vi "Configure Warm Up Supply.vi"(0 "VISA resource name":refnum<visa-resource-name>, 5 "Unpowered Analog Output (3:3)":u16(ring)=3 items=["3"=3, "4"=4], 7 "Warm Up Control  (0:Auto Off)":u16(ring) items=["Auto Off", "Continuous"], 9 "Warm Up Percentage (0.00)":dbl format="%.2f", 11 "error in (no error)":errorcluster) -> (4 "VISA resource name out":refnum<visa-resource-name>, 15 "error out":errorcluster)   [LabVIEW 2019, in "Lake Shore 336.lvlib"]
doc: "This VI configures the Unpowered Analog Output when the mode is set to warm up supply. Warm up supply mode is designed for controlling an external power supply used for rapidly increasing the temperature in order to change samples."
uses:
  Lake Shore 336.lvlib
  Instance           1 32Saved   Configure Warm Up Supply .vi
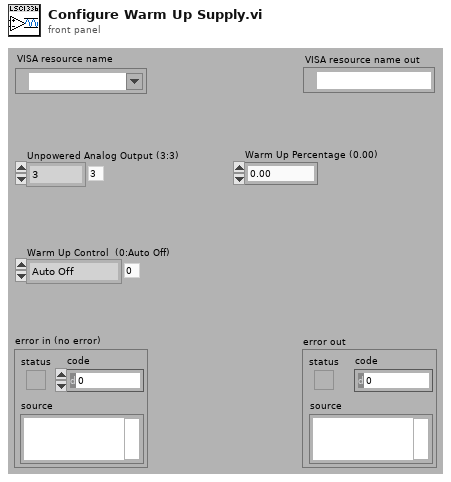
[diagram p1: front panel]
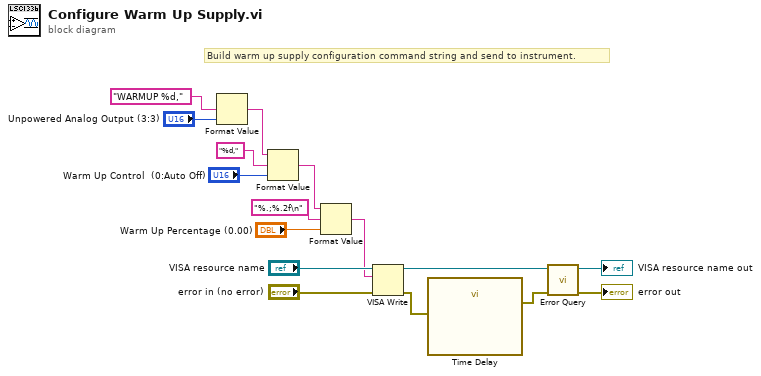
[diagram p0: block diagram]
diagram:
  # "Build warm up supply configuration command string and send to instrument."
  n1 = Format Value(format string="WARMUP %d,", value (0)="Unpowered Analog Output (3:3)") -> (output string=w2:string)  [unwired: 1 in]
  n2 = Format Value(string ("")=w2, format string="%d,", value (0)="Warm Up Control  (0:Auto Off)") -> (output string=w6:string)
  n3 = Format Value(string ("")=w6, format string="%.;%.2f\n", value (0)="Warm Up Percentage (0.00)") -> (output string=w4:string)
  n4 = VISA Write(VISA resource name="VISA resource name", write buffer=w4, error in (no error)="error in (no error)") -> (VISA resource name out=w14:refnum<visa-resource-name>, error out=w11:errorcluster)  [unwired: 1 out]
  n5 = call "Time Delay"("error in (no error)"=w11) -> ("error out"=w10:errorcluster)  [unwired: 10 in]
  n6 = call "Error Query.vi"("error in (no error)"=w10, "VISA resource name"=w14) -> ("error out"=→"error out":errorcluster, "VISA resource name out"=→"VISA resource name out":refnum<visa-resource-name>)  [unwired: 7 in, 1 out]
